vi "Dynamixel XL320 Setup.vi"() -> ()   [LabVIEW 2015]
doc: "This example is designed for configuring attributes typically set on a dynamixel motor before first use."
uses:
  <instrlib>/Dynamixel XL320/Public/Motor Operation/Low Level/XL320_Alarm Setting.ctl
  <instrlib>/Dynamixel XL320/Public/Motor Operation/Low Level/XL320_Baud Setting.ctl
  <instrlib>/Dynamixel XL320/Dynamixel XL320.lvlib
panel:
  out "Current Alarm Settings":cluster{"LED Alarm":T1, "Shutdown Alarm":T1}={"LED Alarm"={"Access"=FALSE, "Angle Limit"=FALSE, "Data Length"=FALSE, "Range"=FALSE, "Checksum"=FALSE, "Instruction"=FALSE, "Result Fail"=FALSE}, "Shutdown Alarm"={"Access"=TRUE, "Angle Limit"=FALSE, "Data Length"=FALSE, "Range"=FALSE, "Checksum"=FALSE, "Instruction"=FALSE, "Result Fail"=FALSE}}
  in  "Desired Alarm Settings":cluster{"LED Alarm":T1, "Shutdown Alarm":T1}
  out "Searching for motor":bool
  in  "Tab Control":enum32{"Port setup", "Auto-detect settings"}(tab)
  in  "VISA resource name":refnum<visa-resource-name>
  in  "Force Baud Rate (True)":bool
  in  "Baud rate (1,000,000 bps)":T2=3 items=["9600 bps", "57600 bps", "115200 bps", "1,000,000 bps"]
  in  "Search Timeout (10000 ms)":u32=10000
  in  "Starting ID (0)":u8
  in  "Ending ID (252)":u8=252
  in  "stop":bool
  out "Current angles":cluster{dbl, dbl, dbl}(knob)={0.0, 0.0, 300.0} scale=0.0..300.0
  in  "Counter-Clockwise Limit":dbl=300.0
  in  "Clockwise Limit":dbl
  out "Current Safety Limits":T3={"Temperature Limit (C)"=80, "Low Voltage Limit (V)"=6.0, "High Voltage Limit (V)"=19.0, "Maximum Torque%"=100.0} {"Maximum Torque%" min=0.0 max=100.0; "High Voltage Limit (V)" min=5.0 max=25.0; "Low Voltage Limit (V)" min=5.0 max=25.0; "Temperature Limit (C)" max=150 step=1}
  in  "Desired Safety Limits":T3={"Temperature Limit (C)"=65, "Low Voltage Limit (V)"=6.0, "High Voltage Limit (V)"=9.0, "Maximum Torque%"=100.0} {"Maximum Torque%" min=0.0 max=100.0; "High Voltage Limit (V)" min=5.0 max=25.0; "Low Voltage Limit (V)" min=5.0 max=25.0; "Temperature Limit (C)" max=150 step=1}
  in  "Apply new settings":bool
  in  "Change ID":bool
  out "Current ID":u8
  in  "New ID":u8
  # "Ghislain REMY, IUT de Cachan, 2015 December 2015"
  # "This example is designed for \nconfiguring attributes typically set \non a Dynamixel motor before first \nuse.  \n\n1. Connect only one motor to the\nserial communications line. \n2. Choose the serial communication \nsettings and optionally the auto \ndetect settings.  \n3. Run the VI.\n4. Change the ID if desired.\n5. Enter other desired settings and\nclick Apply new settings.\n6. Stop the VI and repeat for each\nmotor you wish to configure."
  # "Clockwise Limit"
  # "Motor Position"
  # "Counter-Clockwise Limit"
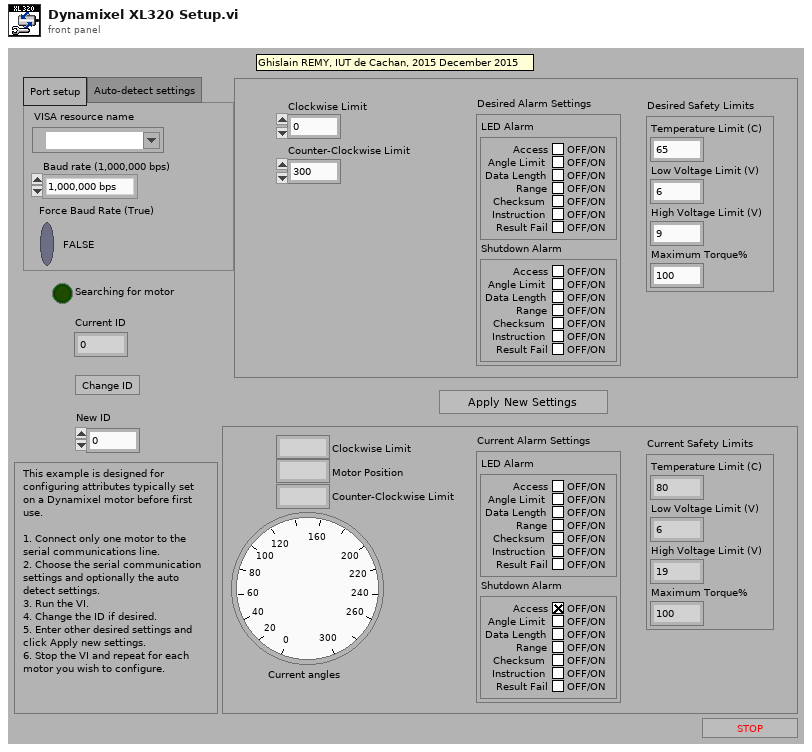
[diagram p1: front panel]
types:
  T1 = typedef "Dynamixel XL320.lvlib/XL320_Alarm Setting.ctl" = cluster{"Access":bool, "Angle Limit":bool, "Data Length":bool, "Range":bool, "Checksum":bool, "Instruction":bool, "Result Fail":bool}
  T2 = typedef "Dynamixel XL320.lvlib/XL320_Baud Setting.ctl" = u8
  T3 = cluster{"Temperature Limit (C)":u8, "Low Voltage Limit (V)":dbl, "High Voltage Limit (V)":dbl, "Maximum Torque%":dbl}
  T4 = cluster{"Boolean array[0]":bool, "Boolean array[1]":bool, "Boolean array[2]":bool, "Boolean array[3]":bool, "Boolean array[4]":bool, "Boolean array[5]":bool, "Boolean array[6]":bool}
  T5 = cluster{"Boolean array":cluster{"Boolean array[0]":bool, "Boolean array[1]":bool, "Boolean array[2]":bool, "Boolean array[3]":bool, "Boolean array[4]":bool, "Boolean array[5]":bool, "Boolean array[6]":bool}, "Boolean array":cluster{"Boolean array[0]":bool, "Boolean array[1]":bool, "Boolean array[2]":bool, "Boolean array[3]":bool, "Boolean array[4]":bool, "Boolean array[5]":bool, "Boolean array[6]":bool}}
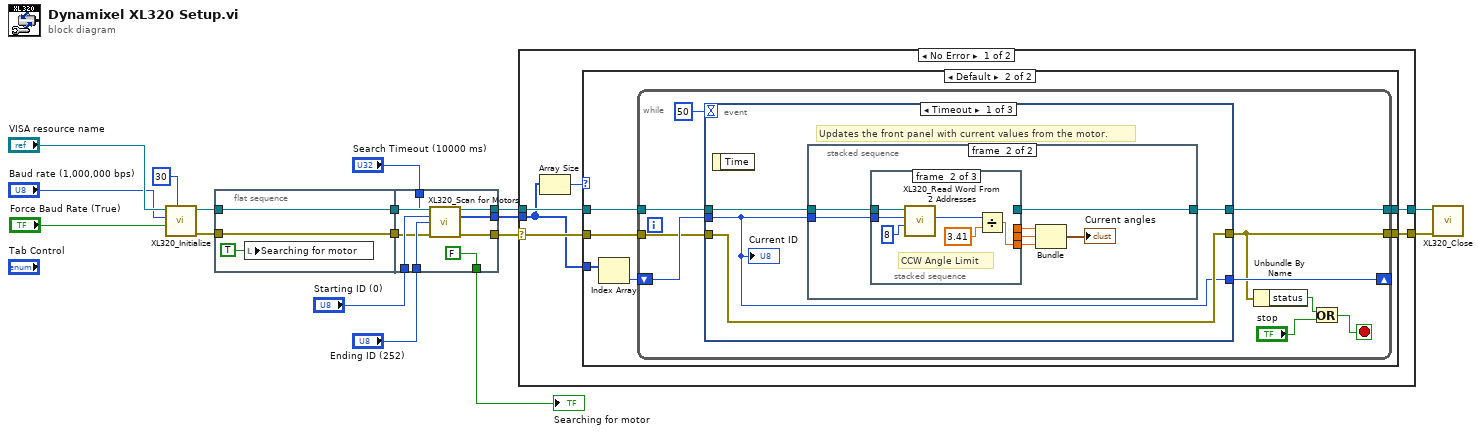
[diagram p0: block diagram]
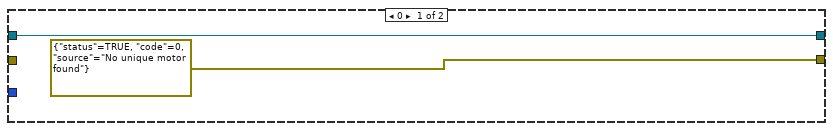
[diagram p2: hidden frame]
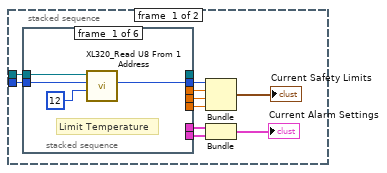
[diagram p3: hidden frame]
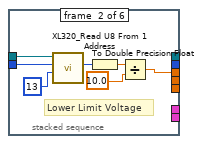
[diagram p4: hidden frame]
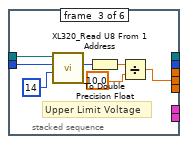
[diagram p5: hidden frame]
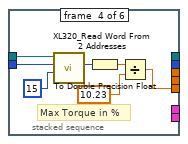
[diagram p6: hidden frame]
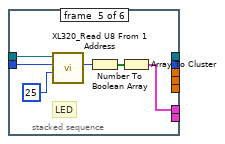
[diagram p7: hidden frame]
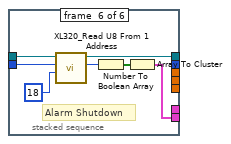
[diagram p8: hidden frame]
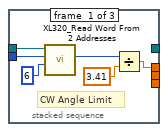
[diagram p9: hidden frame]
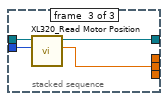
[diagram p10: hidden frame]
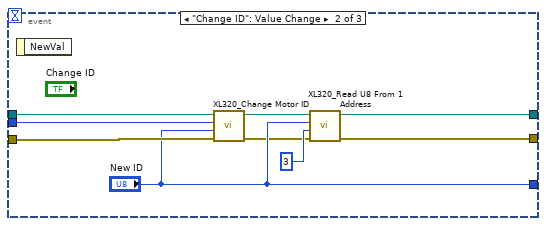
[diagram p11: hidden frame]
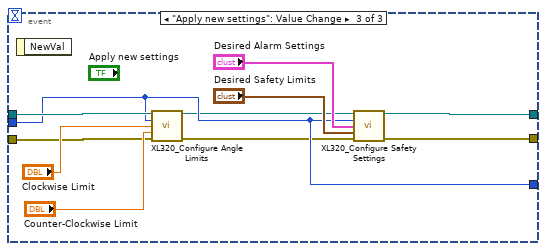
[diagram p12: hidden frame]
diagram:
  n1 = call <instrlib>:"XL320_Initialize.vi"("Timeout (30 msec)"=u32 30 ("timeout (10sec)"), "Force Baud Rate (True)"="Force Baud Rate (True)", "Baud rate (1,000,000 bps)"="Baud rate (1,000,000 bps)", "VISA resource name"="VISA resource name") -> ("error out"=w7:errorcluster, "VISA resource name out"=w8:refnum<visa-resource-name>)  [unwired: 6 in]
  n2 = flat-sequence {
    tunnel: w7 -> [w19]
    tunnel: w8 -> [w20]
    tunnel: [w20] -> w11
    tunnel: [w19] -> w10
    tunnel: [w23] -> w17
    tunnel: [w21] -> w16
    tunnel: [w22] -> w15
    tunnel: "Search Timeout (10000 ms)" -> [w25]
    tunnel: "Starting ID (0)" -> [w27]
    tunnel: "Ending ID (252)" -> [w26]
    tunnel: w11 -> [w28]
    tunnel: w10 -> [w24]
    tunnel: [FALSE ("Searching for motor")] -> w9
    frame #0 {
      n3 = local write "Searching for motor"(TRUE ("Searching for motor")) -> ()
    }
    frame #1 {
      n4 = call <instrlib>:"XL320_Scan for Motors.vi"("VISA resource name"=w28, "Starting ID (0)"=w27, "Ending ID (252)"=w26, "Search Timeout (10000 ms)"=w25, "error in (no error)"=w24) -> ("VISA resource name out"=w23:refnum<visa-resource-name>, "Motors IDs Found"=w22:u8[], "error out"=w21:errorcluster)  [unwired: 8 in]
    }
  }
  n5 = case shown="No Error" w16 {
    selector: w16 -> [w33 w149]
    tunnel: [w35 w150] -> w3
    tunnel: w17 -> [w34 w150]
    tunnel: [w32 w149] -> w2
    tunnel: w15 -> [w31 _]
    frame No Error {
      n6 = Array Size(array=w31) -> (size(s)=w30:i32)
      n7 = case shown="Default" w30 {
        tunnel: [w37 w43] -> w35
        tunnel: w34 -> [w37 w42]
        tunnel: w33 -> [_ w41]
        tunnel: w31 -> [_ w40]
        tunnel: [errorcluster {"status"=TRUE, "code"=0, "source"="No unique motor found"} ("error out") w38] -> w32
        frame 0 {
        }
        frame Default {
          n8 = Index Array(array=w40) -> (element=w39:u8)  [unwired: 1 in]
          n9 = while {
            tunnel: w41 -> [w49]
            shift-right: [w48] -> _
            shift-left: w39 -> [w51]
            tunnel: w42 -> [w52]
            tunnel: [w50] -> w43
            tunnel: [w47] -> w38
            stop <- w46 stop-if-true
            n10 = event shown="[0] Timeout" {
              selector: _ -> [_ _ _]
              dyn-events: _ -> [_ _ _]
              timeout: 50 -> [_ _ _]
              tunnel: w52 -> [w57 w137 w144]
              tunnel: w51 -> [w54 w136 w143]
              tunnel: [w56 w129 w146] -> w50
              tunnel: w49 -> [w55 w135 w140]
              tunnel: [w55 w130 w145] -> w47
              tunnel: [w54 "New ID" w143] -> w48
              event Timeout {
                # "Updates the front panel with current values from the motor."
                n11 = event-data() -> ()  [unwired: 1 in, 1 out]
                n12 = stacked-sequence {
                  tunnel: w57 -> [w66 w108]
                  tunnel: w54 -> [w59 w107]
                  tunnel: [_ w106] -> w56
                  frame #0 {
                    n13 = stacked-sequence {
                      tunnel: w66 -> [w71 w76 w79 w89 w96 w103]
                      tunnel: [w68 _ _ _ _ _] -> w65
                      tunnel: [_ w72 _ _ _ _] -> w64
                      tunnel: [_ _ w83 _ _ _] -> w63
                      tunnel: [_ _ _ w90 _ _] -> w62
                      tunnel: [_ _ _ _ w97 _] -> w61
                      tunnel: [_ _ _ _ _ w104] -> w60
                      tunnel: w59 -> [w70 w75 w80 w88 w95 w102]
                      tunnel: [_ _ _ _ _ w101] -> _
                      frame #0 {
                        # "Limit Temperature"
                        n14 = call <instrlib>:"XL320_Read U8 From 1 Address.vi"("Address number (0)"=u16 12 ("Address # DEC"), "Motor ID (0)"=w70, "VISA resource name"=w71) -> ("Data"=w68:u8)  [unwired: 6 in, 2 out]
                      }
                      frame #1 {
                        # "Lower Limit Voltage"
                        n15 = call <instrlib>:"XL320_Read U8 From 1 Address.vi"("Address number (0)"=u16 13 ("Address # DEC"), "Motor ID (0)"=w75, "VISA resource name"=w76) -> ("Data"=w73:u8)  [unwired: 6 in, 2 out]
                        n16 = To Double Precision Float(number=w73) -> (double precision float=w78:dbl)
                        n17 = Divide(x=w78, y=10.0) -> (x/y=w72:dbl)
                      }
                      frame #2 {
                        # "Upper Limit Voltage"
                        n18 = call <instrlib>:"XL320_Read U8 From 1 Address.vi"("Address number (0)"=u16 14 ("Address # DEC"), "Motor ID (0)"=w80, "VISA resource name"=w79) -> ("Data"=w82:u8)  [unwired: 6 in, 2 out]
                        n19 = To Double Precision Float(number=w82) -> (double precision float=w85:dbl)
                        n20 = Divide(x=w85, y=10.0) -> (x/y=w83:dbl)
                      }
                      frame #3 {
                        # "Max Torque in %"
                        n21 = call <instrlib>:"XL320_Read Word From 2 Addresses.vi"("Address number (0)"=u16 15 ("Address # DEC"), "Motor ID (0)"=w88, "VISA resource name"=w89) -> ("Data"=w87:u16)  [unwired: 6 in, 2 out]
                        n22 = To Double Precision Float(number=w87) -> (double precision float=w92:dbl)
                        n23 = Divide(x=w92, y=10.23) -> (x/y=w90:dbl)
                      }
                      frame #4 {
                        # "LED"
                        n24 = call <instrlib>:"XL320_Read U8 From 1 Address.vi"("Address number (0)"=u16 25 ("Address # DEC"), "Motor ID (0)"=w95, "VISA resource name"=w96) -> ("Data"=w94:u8)  [unwired: 6 in, 2 out]
                        n25 = Number To Boolean Array(number=w94) -> (Boolean array=w98:bool[])
                        n26 = Array To Cluster(array=w98) -> (cluster=w97:T4)
                      }
                      frame #5 {
                        # "Alarm Shutdown"
                        n27 = call <instrlib>:"XL320_Read U8 From 1 Address.vi"("Address number (0)"=u16 18 ("Address # DEC"), "Motor ID (0)"=w102, "VISA resource name"=w103) -> ("Data"=w100:u8, "VISA resource name out"=w101:refnum<visa-resource-name>)  [unwired: 6 in, 1 out]
                        n28 = Number To Boolean Array(number=w100) -> (Boolean array=w105:bool[])
                        n29 = Array To Cluster(array=w105) -> (cluster=w104:T4)
                      }
                    }
                    n30 = Bundle("Data"=w65, w64, w63, w62) -> (→"Current Safety Limits":cluster{"Data":u8, dbl, dbl, dbl})  [unwired: 1 in]
                    n31 = Bundle("Boolean array"=w61, "Boolean array"=w60) -> (→"Current Alarm Settings":T5)  [unwired: 1 in]
                  }
                  frame #1 {
                    n32 = stacked-sequence {
                      tunnel: w108 -> [w116 w122 w128]
                      tunnel: w107 -> [w115 w121 w127]
                      tunnel: [w117 _ _] -> w111
                      tunnel: [_ _ w126] -> w110
                      tunnel: [_ w123 _] -> w109
                      tunnel: [_ _ w125] -> w106
                      frame #0 {
                        # "CW Angle Limit"
                        n33 = call <instrlib>:"XL320_Read Word From 2 Addresses.vi"("Address number (0)"=u16 6 ("Address # DEC"), "Motor ID (0)"=w115, "VISA resource name"=w116) -> ("Data"=w114:u16)  [unwired: 6 in, 2 out]
                        n34 = Divide(x=w114, y=3.41) -> (x/y=w117:dbl)
                      }
                      frame #1 {
                        # "CCW Angle Limit"
                        n35 = call <instrlib>:"XL320_Read Word From 2 Addresses.vi"("Address number (0)"=u16 8 ("Address # DEC"), "Motor ID (0)"=w121, "VISA resource name"=w122) -> ("Data"=w119:u16)  [unwired: 6 in, 2 out]
                        n36 = Divide(x=w119, y=3.41) -> (x/y=w123:dbl)
                      }
                      frame #2 {
                        n37 = call <instrlib>:"XL320_Read Motor Position.vi"("Motor ID (0)"=w127, "VISA resource name"=w128) -> ("Position (deg)"=w126:dbl, "VISA resource name out"=w125:refnum<visa-resource-name>)  [unwired: 7 in, 1 out]
                      }
                    }
                    n38 = Bundle(w111, "Position (deg)"=w110, w109) -> (→"Current angles":cluster{dbl, "Position (deg)":dbl, dbl})  [unwired: 1 in]
                  }
                }
                "Current ID" <- w54
              }
              event "Change ID": Value Change {
                n39 = event-data() -> ()  [unwired: 1 in, 1 out]
                n40 = call <instrlib>:"XL320_Change Motor ID.vi"("error in (no error)"=w135, "New ID"="New ID", "Current ID"=w136, "VISA resource name"=w137) -> ("error out"=w131:errorcluster, "VISA Resource Out"=w134:refnum<visa-resource-name>)  [unwired: 6 in]
                n41 = call <instrlib>:"XL320_Read U8 From 1 Address.vi"("Error in (no error)"=w131, "Address number (0)"=u16 3 ("Address number (dec)"), "Motor ID (0)"="New ID", "VISA resource name"=w134) -> ("error out"=w130:errorcluster, "VISA resource name out"=w129:refnum<visa-resource-name>)  [unwired: 5 in, 1 out]
              }
              event "Apply new settings": Value Change {
                n42 = event-data() -> ()  [unwired: 1 in, 1 out]
                n43 = call <instrlib>:"XL320_Configure Angle Limits.vi"("VISA resource name"=w144, "Motor ID (0)"=w143, "Clockwise Angle Limit (0 deg)"="Clockwise Limit", "Counter-Clockwise Angle Limit (300 deg)"="Counter-Clockwise Limit", "error in (no error)"=w140) -> ("VISA resource name out"=w138:refnum<visa-resource-name>, "error out"=w139:errorcluster)  [unwired: 9 in]
                n44 = call <instrlib>:"XL320_Configure Safety Settings.vi"("VISA resource name"=w138, "Motor ID (0)"=w143, "Alarm Settings"="Desired Alarm Settings", "Safety Limits"="Desired Safety Limits", "error in (no error)"=w139) -> ("VISA resource name out"=w146:refnum<visa-resource-name>, "error out"=w145:errorcluster)  [unwired: 9 in]
              }
            }
            n45 = Unbundle By Name(w47) -> ("status"=w45:bool)
            n46 = Or(x=w45, y="stop") -> (x .or. y?=w46:bool)
          }
        }
      }
    }
    frame Error {
    }
  }
  n47 = call <instrlib>:"XL320_Close.vi"("error in (no error)"=w2, "VISA resource name"=w3) -> ()  [unwired: 9 in, 1 out]
  "Searching for motor" <- w9
